vi "SetAxisHomePosition.vi"(8 "error in (no error)":errorcluster, 10 "HomePosition":i32, 11 "Picomoto8742ControllerClass in":refnum<class "Picomoto8742ControllerClass.lvclass">) -> (0 "error out":errorcluster, 2 "Success?":bool, 3 "Picomoto8742ControllerClass out":refnum<class "Picomoto8742ControllerClass.lvclass">)   [LabVIEW 2013, in "Picomoto8742ControllerClass.lvclass"]
doc: "Send the home position setting relative to the active axis, to the physical device"
uses:
  Picomoto8742ControllerClass.lvclass
  Picomoto8742ControllerClass.lvclass/Picomoto8742ControllerClass.ctl
  Picomotor8742Axis.lvclass
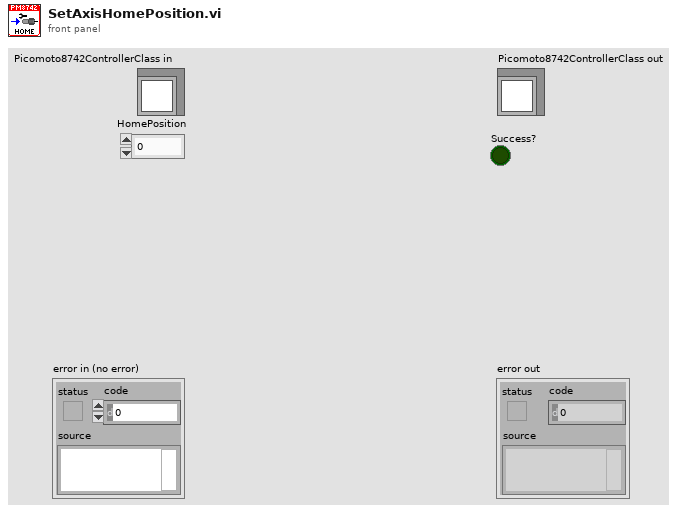
[diagram p1: front panel]
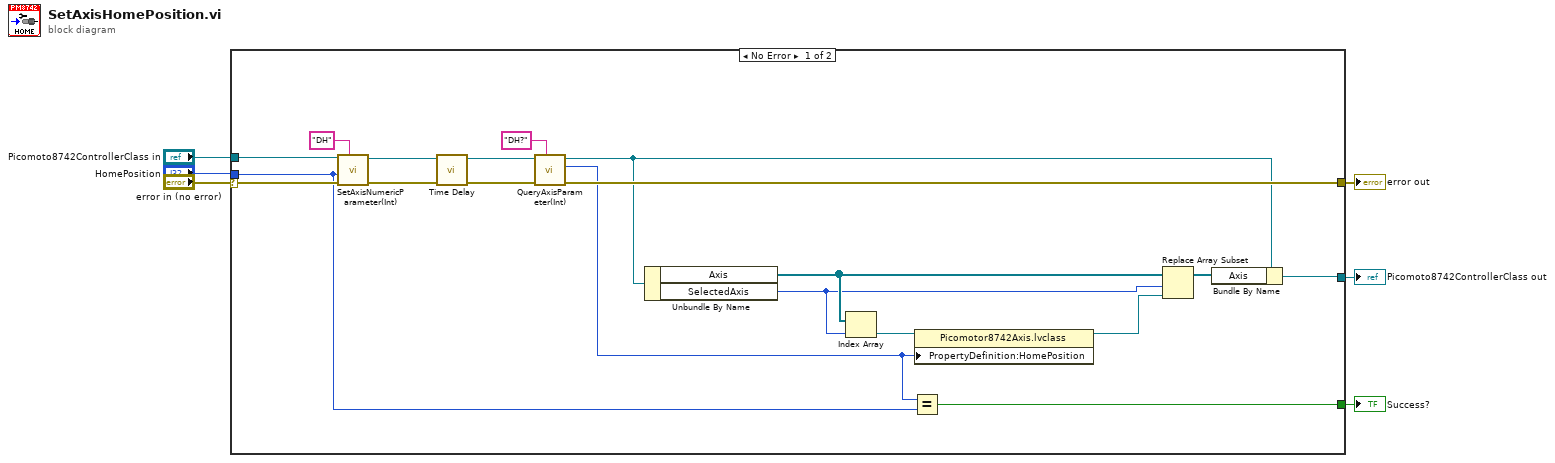
[diagram p0: block diagram]
diagram:
  n1 = case shown="No Error" "error in (no error)" {
    selector: "error in (no error)" -> [w23 w26]
    tunnel: [w22 w26] -> w5
    tunnel: [w19 w25] -> w3
    tunnel: "Picomoto8742ControllerClass in" -> [w18 w25]
    tunnel: "HomePosition" -> [w8 _]
    tunnel: [w7 _] -> w1
    frame No Error {
      n2 = call "SetAxisNumericParameter(Int).vi"("CMD"="DH" ("string"), "error in (no error)"=w23, "ParameterValue"=w8, "Picomoto8742ControllerClass in"=w18) -> ("error out"=w24:errorcluster, "Picomoto8742ControllerClass Out"=w15:refnum<class "Picomoto8742ControllerClass.lvclass">)  [unwired: 6 in]
      n3 = call "Time Delay"("error in (no error)"=w24) -> ("error out"=w10:errorcluster)  [unwired: 10 in]
      n4 = call-dynamic "QueryAxisParameter(Int).vi"("Cmd"="DH?" ("string"), "error in (no error)"=w10, "Picomoto8742ControllerClass in"=w15) -> ("error out"=w22:errorcluster, "ValueOut"=w9:i32, "Picomoto8742ControllerClass Out"=w11:refnum<class "Picomoto8742ControllerClass.lvclass">)  [unwired: 6 in]
      n5 = Unbundle By Name(w11) -> ("Axis"=w14:refnum<class "Picomotor8742Axis.lvclass">[], "SelectedAxis"=w13:u32)
      n6 = Index Array(array=w14, index=w13) -> (element=w12:refnum<class "Picomotor8742Axis.lvclass">)
      n7 = Equal?(x=w9, y=w8) -> (x = y?=w7:bool)
      n8 = property class="Picomotor8742Axis.lvclass"(reference=w12, "PropertyDefinition:HomePosition"=w9) -> (reference out=w21:refnum<class "Picomotor8742Axis.lvclass">)  [unwired: 1 in, 1 out]
      n9 = Replace Array Subset(array=w14, new element=w21, index=w13) -> (w20:refnum<class "Picomotor8742Axis.lvclass">[])
      n10 = Bundle By Name(cluster=w11, "Axis"=w20) -> (w19:refnum<class "Picomoto8742ControllerClass.lvclass">)
    }
    frame Error {
    }
  }
  "error out" <- w5
  "Picomoto8742ControllerClass out" <- w3
  "Success?" <- w1
